vi "SERIAL_DecodeYPRUpdatePacket.vi"(8 "error in":errorcluster, 10 "Buffer":string) -> (0 "error out":errorcluster, 1 "Valid":bool, 2 "YPR Update":T1)   [LabVIEW 2014]
uses:
  COMMON/TypeDefs/Data TypeDefs/navX YPRH Data.ctl
  navX-MXP IMU.lvlib
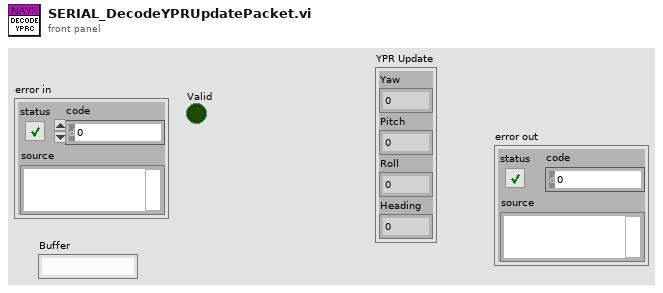
[diagram p1: front panel]
types:
  T1 = typedef "navX-MXP IMU.lvlib/navX YPRH Data.ctl" = cluster{"Yaw":dbl, "Pitch":dbl, "Roll":dbl, "Heading":dbl}
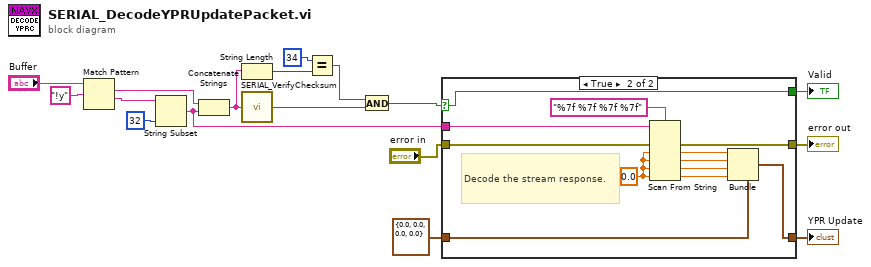
[diagram p0: block diagram]
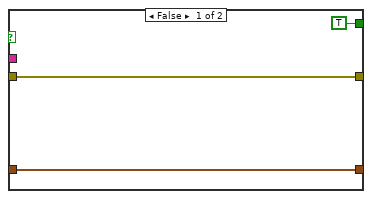
[diagram p2: hidden frame]
diagram:
  n1 = Match Pattern(string="Buffer", regular expression="!y") -> (match substring=w13:string, after substring=w15:string)  [unwired: 1 in, 2 out]
  n2 = String Subset(string=w15, length (rest)=32 ("length (rest)")) -> (substring=w3:string)  [unwired: 1 in]
  n3 = Concatenate Strings(w13, w3) -> (w4:string)
  n4 = String Length(string=w4) -> (length=w9:i32)
  n5 = call "SERIAL_VerifyChecksum.vi"("Content"=w4) -> ("Valid Checksum"=w12:bool)
  n6 = Equal?(x=34, y=w9) -> (x = y?=w7:bool)
  n7 = And(x=w7, y=w12) -> (x .and. y?=w11:bool)
  n8 = case shown="True" w11 {
    selector: w11 -> [_ w25]
    tunnel: [w20 w32] -> w10
    tunnel: w3 -> [_ w31]
    tunnel: "error in" -> [w20 w26]
    tunnel: [TRUE w25] -> w5
    tunnel: T1 {"Yaw"=0.0, "Pitch"=0.0, "Roll"=0.0, "Heading"=0.0} ("YPR Update") -> [w18 w23]
    tunnel: [w18 w22] -> w2
    frame False {
    }
    frame True {
      w24 = 0.0 ("default value 4")
      # "Decode the stream response."
      n9 = Scan From String(format string="%7f %7f %7f %7f", input string=w31, error in=w26, default 1=w24, default 2=w24, default 3=w24, default 4=w24) -> (error out=w32:errorcluster, output 1=w21:dbl, output 2=w29:dbl, output 3=w28:dbl, output 4=w27:dbl)  [unwired: 1 in, 2 out]
      n10 = Bundle(cluster=w23, "Yaw"=w21, "Pitch"=w29, "Roll"=w28, "Heading"=w27) -> (w22:T1)
    }
  }
  "error out" <- w10
  "Valid" <- w5
  "YPR Update" <- w2
